vi "NoLoopEvaluation_sln.vi"(1 "target_input":dbl format="%#_13g", 2 "cal_counter_input":u32) -> (0 "target_output":dbl)   [LabVIEW 2014]
panel:
  # "cal_counter_input : 0\ntarget_input : 1"
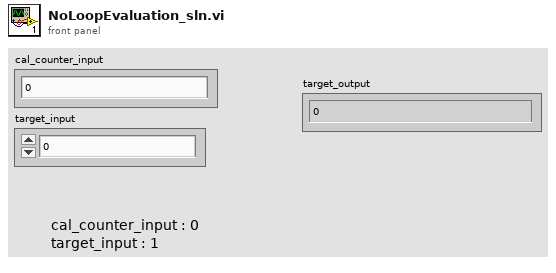
[diagram p1: front panel]
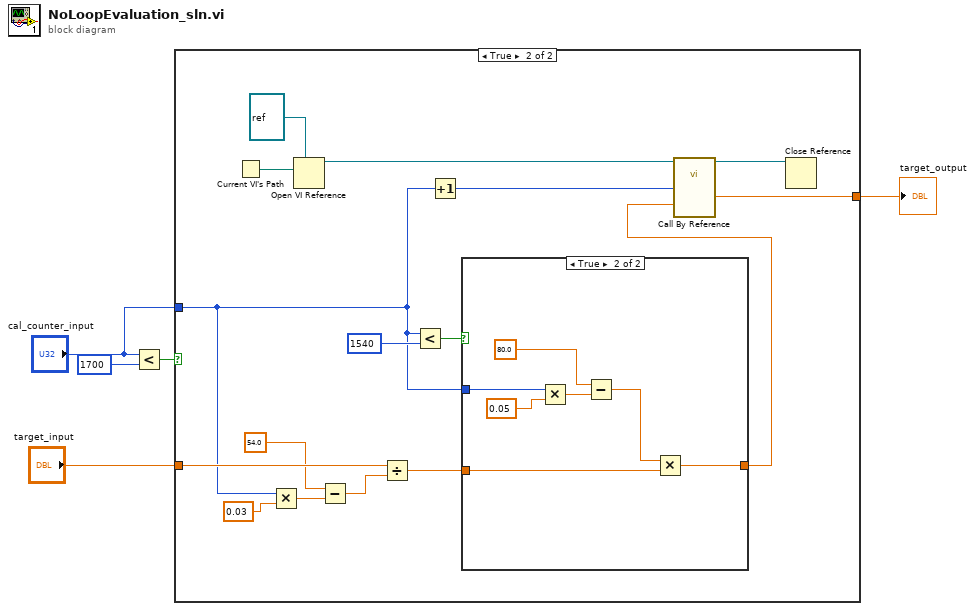
[diagram p0: block diagram]
diagram:
  n1 = Less?(x="cal_counter_input", y=u32 1700) -> (x < y?=w4:bool)
  n2 = case shown="True" w4 {
    tunnel: "target_input" -> [w6 w22]
    tunnel: "cal_counter_input" -> [_ w12]
    tunnel: [w6 w8] -> w1
    frame False {
    }
    frame True {
      n3 = Current VI's Path() -> (path=w14:path)
      n4 = Multiply(x=w12, y=0.03) -> (x*y=w18:dbl)
      n5 = Open VI Reference(type specifier VI Refnum (for type only)=refnum<vi> refnum, vi path=w14) -> (vi reference=w11:refnum<vi>)  [unwired: 4 in, 1 out]
      n6 = Subtract(x=54.0, y=w18) -> (x-y=w16:dbl)
      n7 = Divide(x=w22, y=w16) -> (x/y=w15:dbl)
      n8 = Less?(x=w12, y=u32 1540) -> (x < y?=w21:bool)
      n9 = Increment(x=w12) -> (x+1=w10:u32)
      n10 = case shown="True" w21 {
        tunnel: w15 -> [w23 w26]
        tunnel: w12 -> [_ w30]
        tunnel: [w23 w24] -> w9
        frame False {
        }
        frame True {
          n11 = Multiply(x=w30, y=0.05) -> (x*y=w28:dbl)
          n12 = Subtract(x=80.0, y=w28) -> (x-y=w25:dbl)
          n13 = Multiply(x=w25, y=w26) -> (x*y=w24:dbl)
        }
      }
      n14 = call-by-ref "?"(reference=w11, "target_input"=w9, "cal_counter_input"=w10) -> (reference out=w7:refnum<vi>, "target_output"=w8:dbl)  [unwired: 1 in, 1 out]
      n15 = Close Reference(reference=w7) -> ()  [unwired: 1 in, 1 out]
    }
  }
  "target_output" <- w1
